vi "client.workspace_rid.vi"(8 "error in":errorcluster, 11 "Client in":refnum<class "Client.lvclass">) -> (0 "error out":errorcluster, 3 "Client out":refnum<class "Client.lvclass">)   [LabVIEW 2020, in "Client.lvclass"]
doc: "Returns the workspace the client is connected to, if one was set."
uses:
  Client.lvclass
  client.lvlib
panel:
  out "out_needed out":u32
  out "workspace rid":string
  out "is_present out":bool
  in  "out_needed":u32
  in  "cap":u32
  in  "buf":string
  in  "is_present":bool
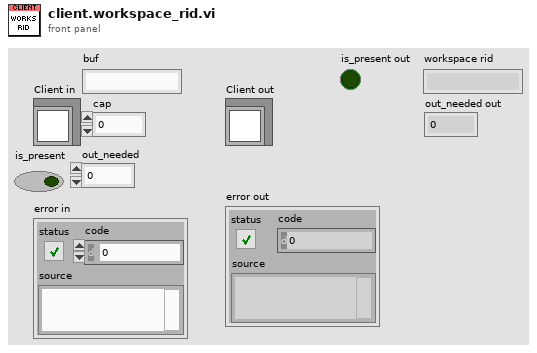
[diagram p1: front panel]
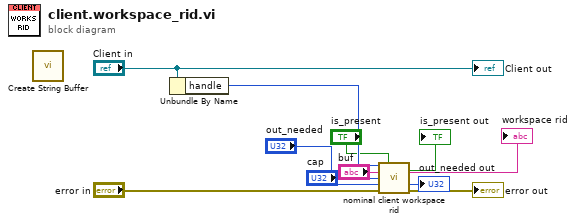
[diagram p0: block diagram]
diagram:
  n1 = call "Create String Buffer.vi"() -> ()  [unwired: 9 in, 3 out]
  n2 = Unbundle By Name("Client in") -> ("handle"=w9:i32)
  n3 = call "nominal client workspace rid.vi"("client"=w9, "is_present"="is_present", "buf"="buf", "cap"="cap", "out_needed"="out_needed", "error in (no error)"="error in") -> ("is_present out"=→"is_present out":bool, "buf out"=→"workspace rid":string, "out_needed out"=→"out_needed out":u32, "error out"=→"error out":errorcluster)  [unwired: 5 in, 1 out]
  "Client out" <- "Client in"
